vi "projekt 1.vi"() -> ()   [LabVIEW 2017]
panel:
  in  "stop":bool
  out "Waveform Graph":dbl[](graph)
  out "temp C":dbl
  out "Waveform Chart":dbl(graph)
  in  "Boolean":bool
  in  "Temp F":dbl(slide) scale=0.0..200.0
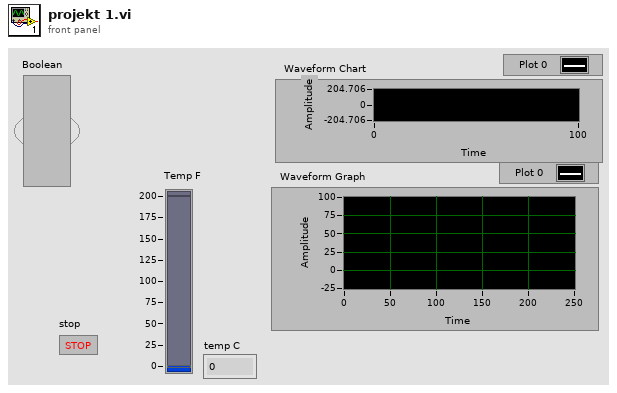
[diagram p1: front panel]
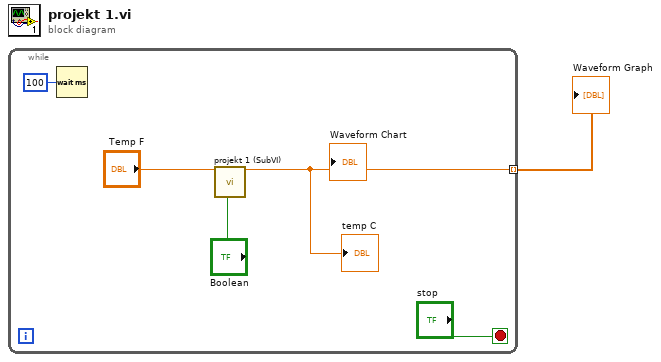
[diagram p0: block diagram]
diagram:
  n1 = while {
    tunnel: [w2] -> w1 mode=indexing
    stop <- "stop" stop-if-true
    n2 = Wait (ms)(milliseconds to wait=u32 100) -> ()  [unwired: 1 out]
    n3 = call "projekt 1 (SubVI).vi"("Temp F"="Temp F", "Boolean"="Boolean") -> ("Numeric Control"=w2:dbl)  [unwired: 17 in]
    "Waveform Chart" <- w2
    "temp C" <- w2
  }
  "Waveform Graph" <- w1
